vi "2B_Tech Serial Data Recording & DECADE 3.1.vi"() -> ()   [LabVIEW 2014]
uses:
  <vilib>/Instr/_visa.llb/VISA Set IO Buffer Mask.ctl
  <vilib>/Instr/_visa.llb/VISA Flush IO Buffer Mask.ctl
  <vilib>/Platform/TimedLoop/XDataNode/timing_clust.ctl
  <vilib>/Platform/TimedLoop/XDataNode/nitl_modes.ctl
  <vilib>/Platform/TimedLoop/XDataNode/wakeup.ctl
  C:/Program Files (x86)/National Instruments/LabVIEW 2014/examples/Data Communication/Network Streams/Simple Network Streams/support/Network Stream Command.ctl
  <vilib>/Utility/error.llb/whitespace.ctl
  <vilib>/Instr/_visa.llb/VISA Configure Serial Port (Instr).vi
  <vilib>/Utility/tcp.llb/UDP Multicast Write-Only Open.vi
  <vilib>/platform/TimedLoop/XDataNode/XDataNode.xnode
  <vilib>/Platform/TimedLoop/XDataNode/XDNodeRunTimeDep.lvlib
panel:
  out "SEPTIC TCP Error Out":errorcluster
  out "TCP packet\nSend to SEPTIC":bool
  in  "stop 2":bool
  out "FISH TCP Error Out":errorcluster
  out "TCP packet\nSend to FISH":bool
  in  "stop":bool
  out "Default file name":string
  out "error out":errorcluster
  out "Ambient/Cabin":bool
  out "Stop File Write":bool
  in  "timeout (10sec)":u32=3000
  in  "VISA resource name":refnum<visa-resource-name>="ASRL2::INSTR"
  out "Simulate 3 av":dbl
  out "Simulate\nConc":i32
  out "Simulate\nconc":bool
  out "3hr_alm_thresh":i32=80
  out "3hrAvg_Alarm":bool
  out "Inst_Alarm":bool
  out "Inst_alm_thresh":i32=220
  out "Time":string
  in  "Clear Display\nErrors":bool
  out "Read Error Counter\nfrom process loop":u32
  out "CABOZO UDP_ASCII_Out":string
  out "Ozo_array":string[](array[string])
  out "3hr_ozo_avg":dbl
  out "q_size":i32
  out "Data Output":string[](array[string])
  out "UDP packet\nSend status":bool
  out "TWBOZO UDP_ASCII_Out":string
  out "UDP_Out_Error":errorcluster
  out "UDP_Pack_num":u32
  out "Flight Number":string
  out "Number of times \nRead time out":u32
  out "Data Loop count":i32
  out "2B_Serial_error out":errorcluster
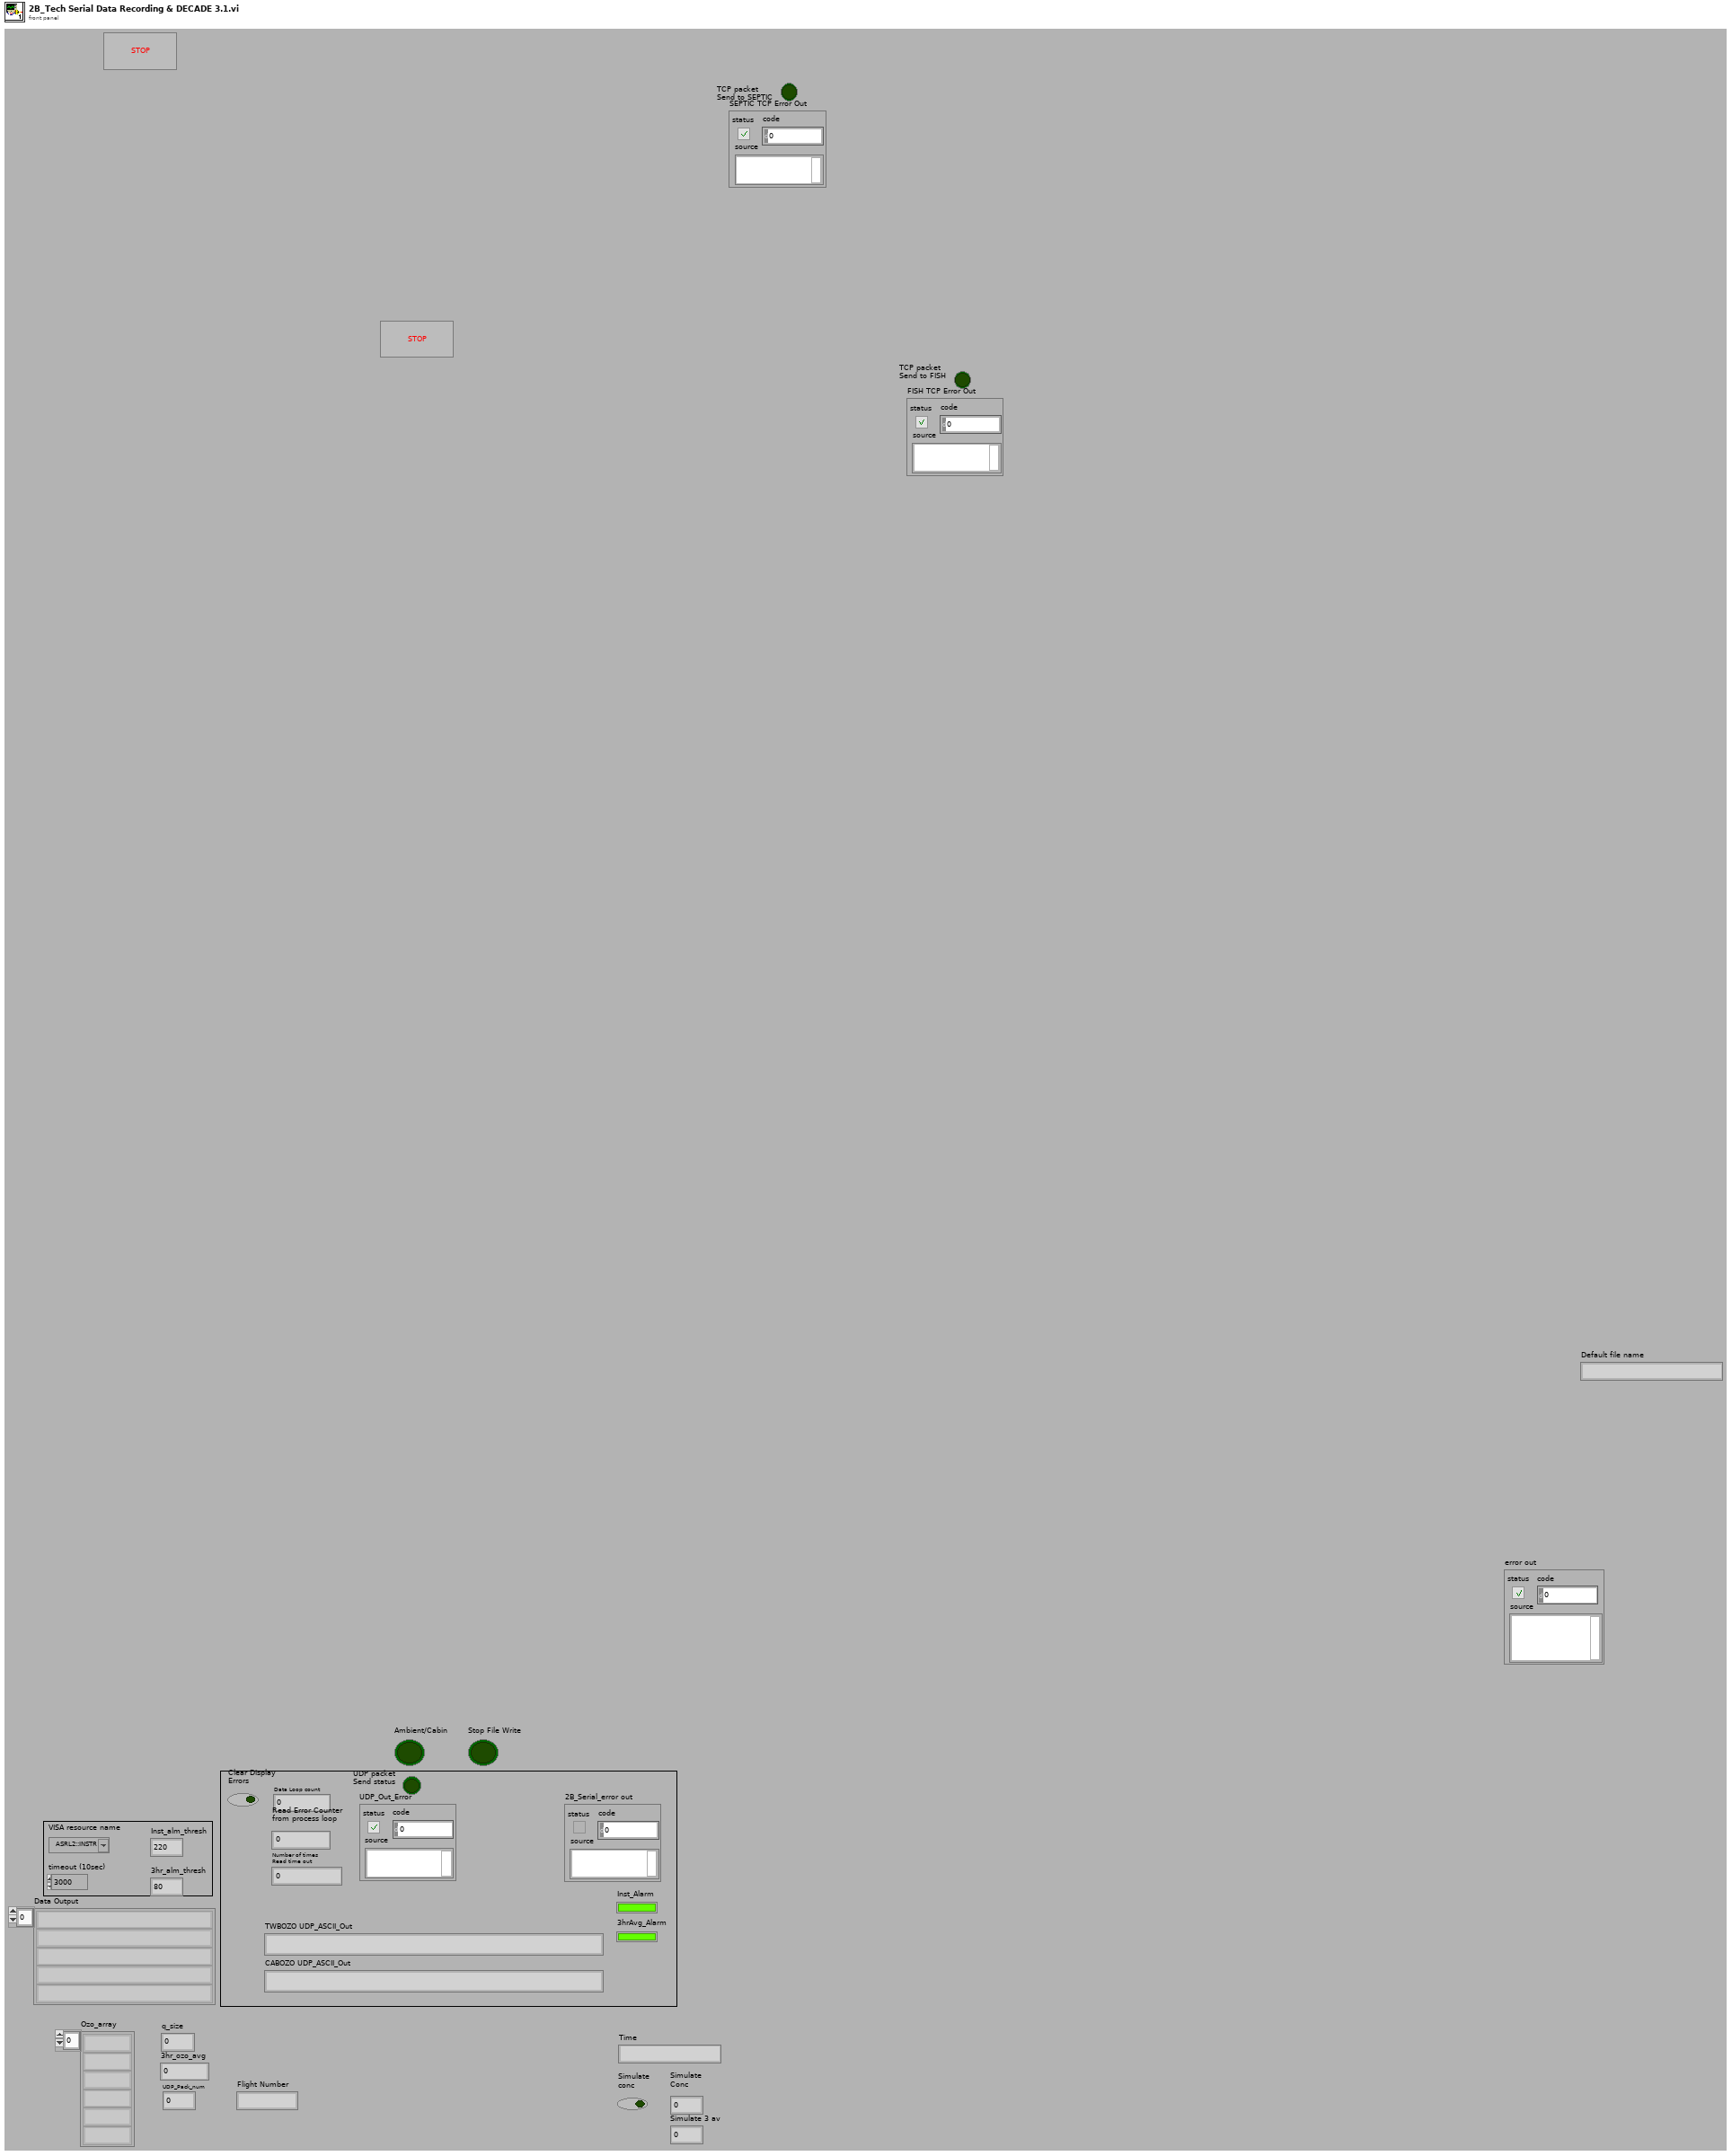
[diagram p1: front panel]
types:
  T1 = typedef "VISA Flush IO Buffer Mask.ctl" = u16
  T2 = typedef "VISA Set IO Buffer Mask.ctl" = u16
  T3 = typedef "XDNodeRunTimeDep.lvlib/timing_clust.ctl" = cluster{"Expected End [f-1]":u64, "Actual End [f-1]":u64, "Finished Late? [f-1]":bool, "Expected End [i-1]":u64, "Actual End [i-1]":u64, "Finished Late? [i-1]":bool, "Expected Start [i]":u64, "Actual Start [i]":u64, "Expected Start [f]":u64, "Actual Start [f]":u64, "Source Name":string, "Structure Name":string, "Period":i64, "Deadline":i64, "Offset":i64, "Start":i64, "Priority":i32, "Timeout":i32, "Mode":T4, "Wakeup Reason":T5, "Error":errorcluster, "Source Type":string, "Secondary Source Type":string, "Global End Time":u64, "Global Start Time":u64, "Frame Duration":u64, "Iteration Duration":u64, "Assigned CPU":i32, "I/O Scan Engine Mode":u32}
  T4 = typedef "XDNodeRunTimeDep.lvlib/nitl_modes.ctl" = enum32{"No Change", "Process missed periods, maintain original phase", "Discard missed periods, maintain original phase", "Process missed periods, ignore original phase", "Discard missed periods, ignore original phase"}
  T5 = typedef "XDNodeRunTimeDep.lvlib/wakeup.ctl" = enum32{"Normal", "Aborted", "Asynchronous wakeup", "Timing source error", "Timed loop error", "Timeout"}
  T6 = typedef "Network Stream Command.ctl" = cluster{"Message":string, "Message Data":variant}
  T7 = enum16{"open", "replace", "create", "open or create", "replace or create", "replace or create with confirmation"}
  T8 = typedef "whitespace.ctl" = u16
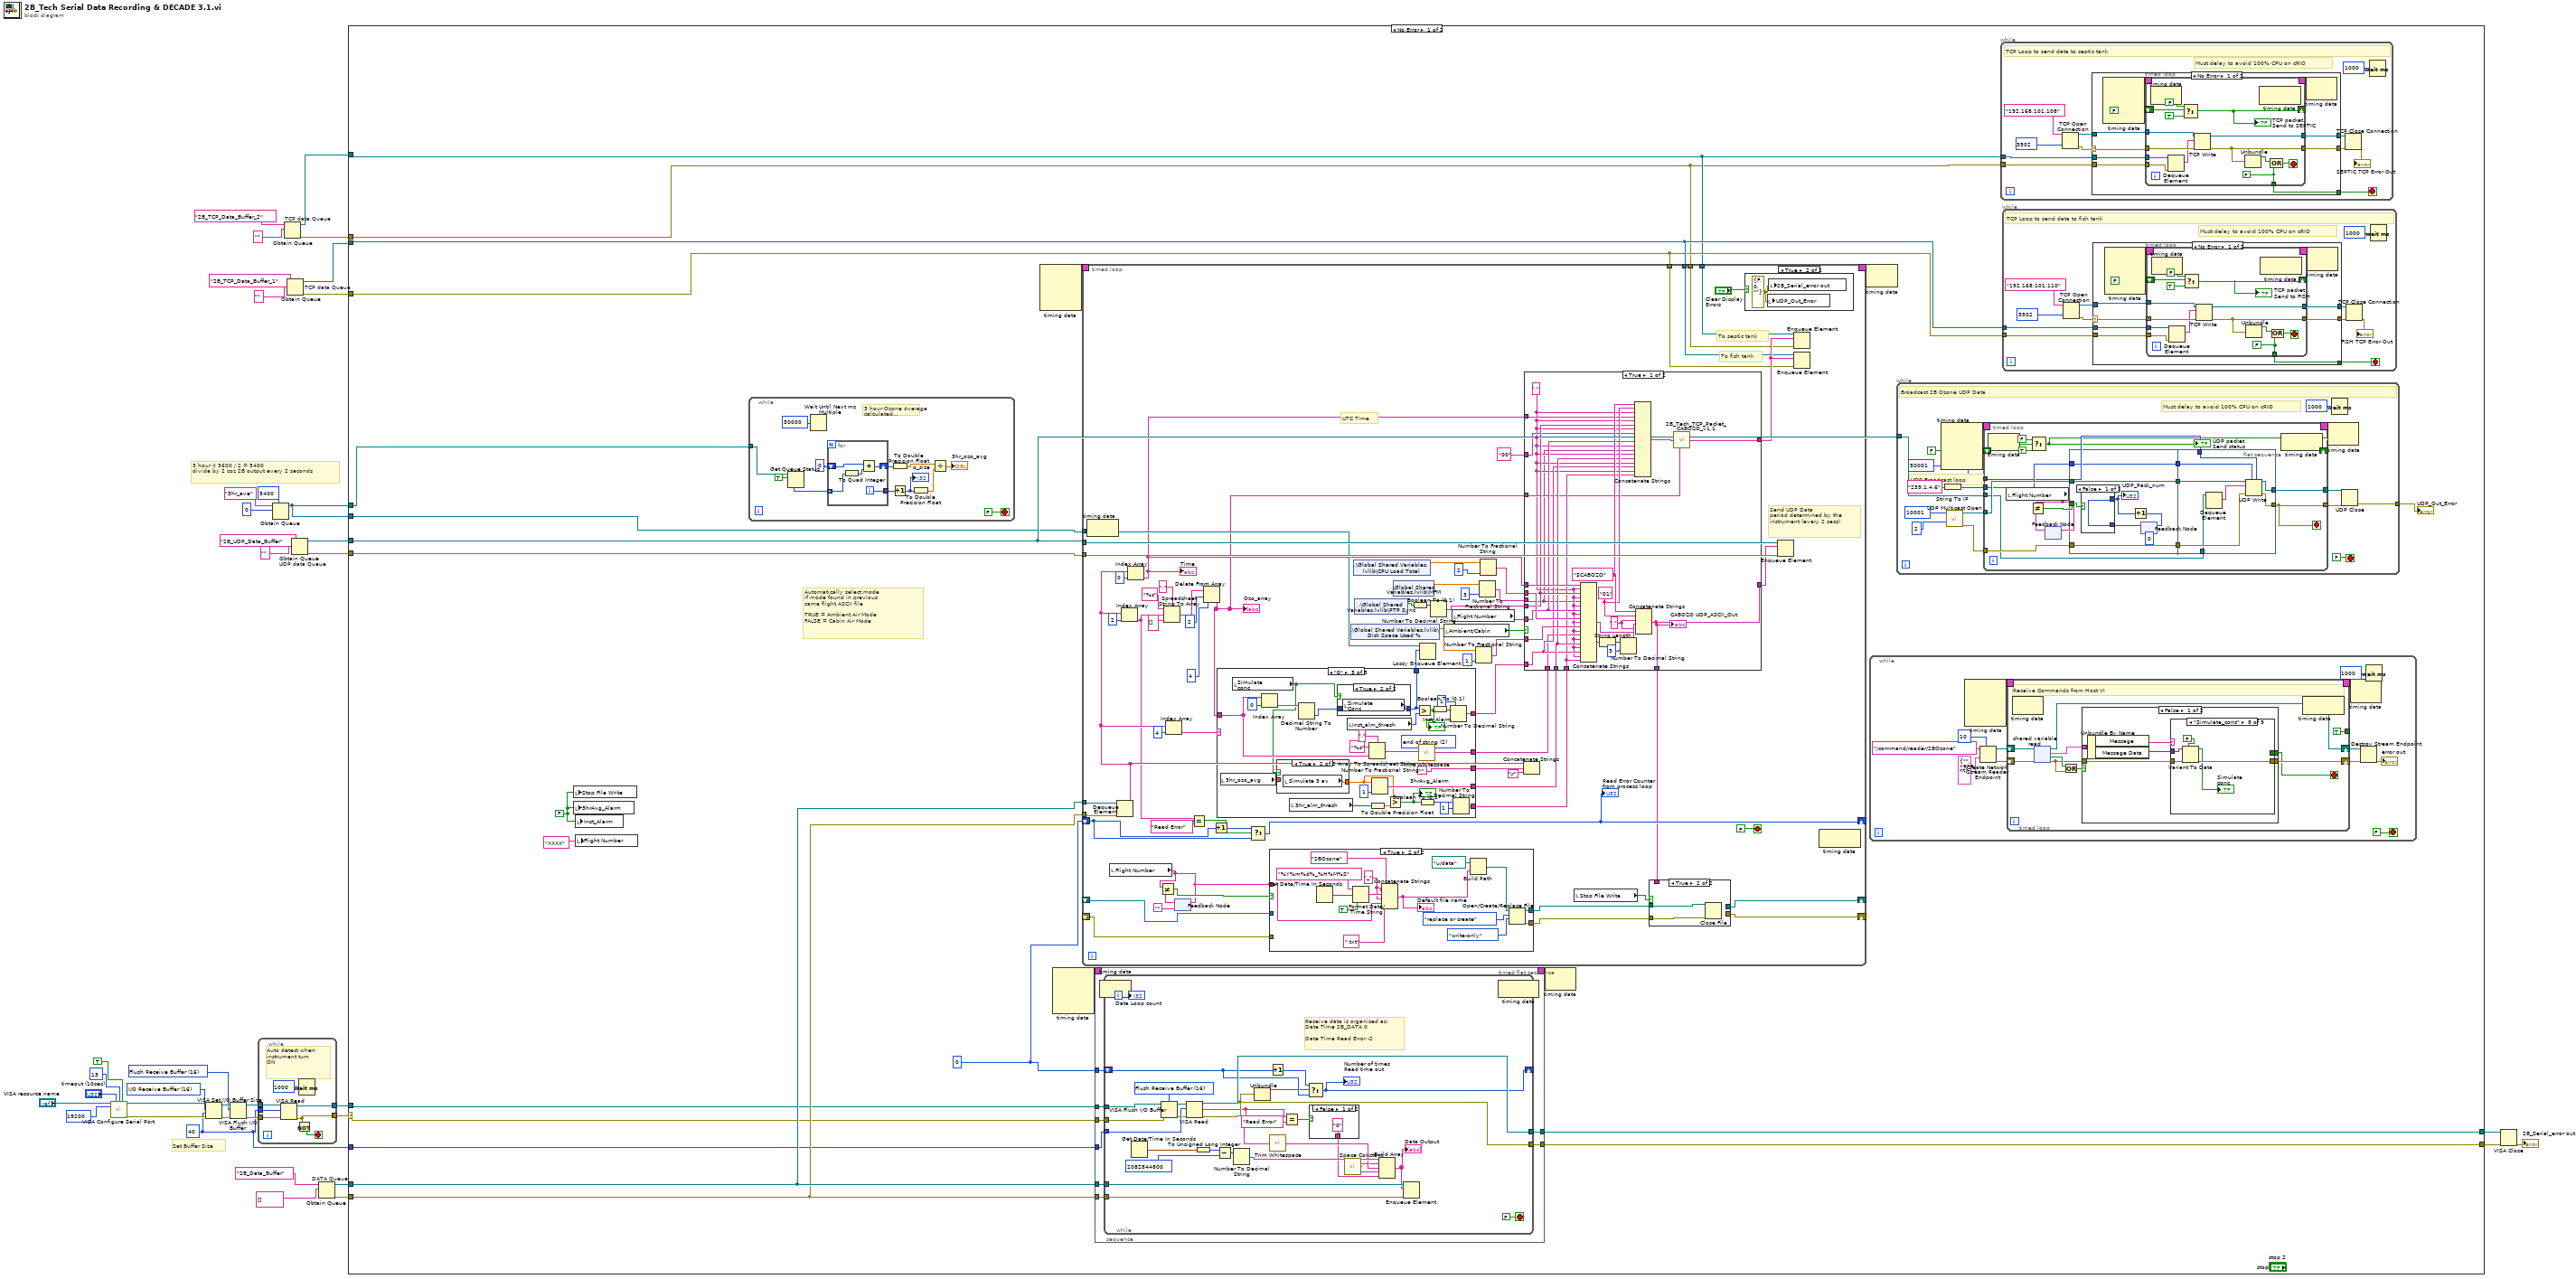
[diagram p0: block diagram]
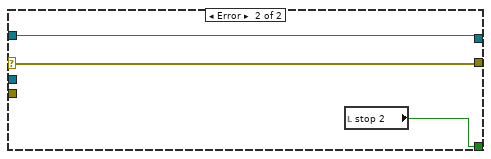
[diagram p2: hidden frame]
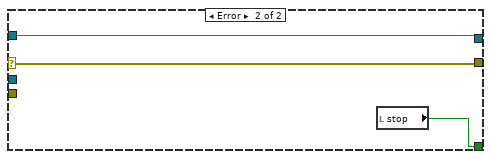
[diagram p3: hidden frame]
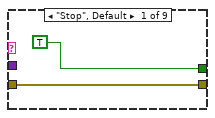
[diagram p4: hidden frame]
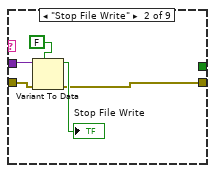
[diagram p5: hidden frame]
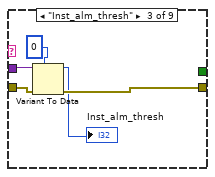
[diagram p6: hidden frame]
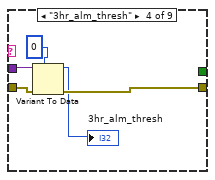
[diagram p7: hidden frame]
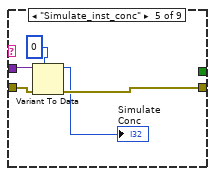
[diagram p8: hidden frame]
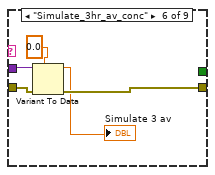
[diagram p9: hidden frame]
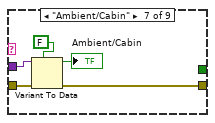
[diagram p10: hidden frame]
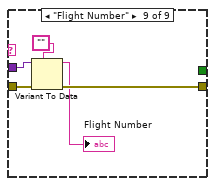
[diagram p11: hidden frame]
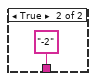
[diagram p13: hidden frame]
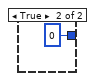
[diagram p14: hidden frame]
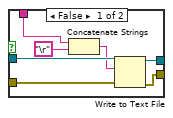
[diagram p15: hidden frame]
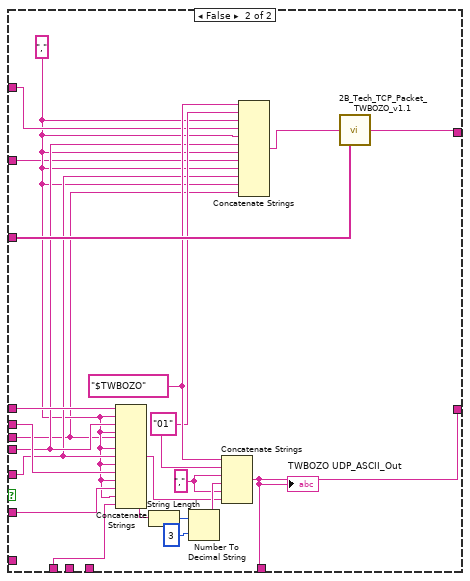
[diagram p18: hidden frame]
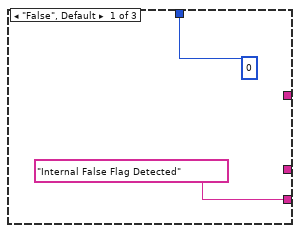
[diagram p19: hidden frame]
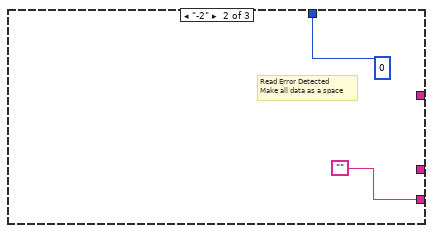
[diagram p20: hidden frame]
diagram:
  w9 = u32 40 ("size (4096)")
  w16 = T1 16 items=["Flush Receive Buffer"=16, "Write Transmit Buffer to Device"=32, "Flush Receive Buffer (No I/O)"=64, "Flush Transmit Buffer"=128] ("Mask")
  w17 = T2 16 items=["I/O Receive Buffer"=16, "I/O Transmit Buffer"=32, "I/O Receive and Transmit Buffer"=48] ("Mask")
  # "Set Buffer Size"
  # "3 hour X 3600 / 2 = 5400\ndivide by 2 coz 2B output every 2 seconds"
  n1 = call-poly "VISA Configure Serial Port"("VISA resource name"="VISA resource name", "timeout (10sec)"="timeout (10sec)", "termination char\n(0xA = '\\n' = LF)"=u8 13 ("termination char\n(0xA = '\\n' = LF)"), "Enable Termination\nChar (T)"=TRUE ("Enable Termination\nChar (T)"), "baud rate (9600)"=u32 19200) -> ("VISA resource name out"=w15:refnum<visa-resource-name>, "error out"=w14:errorcluster)  [unwired: 9 in]
  n2 = VISA Set I/O Buffer Size(VISA resource name=w15, mask (16)=w17, size (4096)=w9, error in (no error)=w14) -> (VISA resource name out=w18:refnum<visa-resource-name>, error out=w19:errorcluster)
  n3 = VISA Flush I/O Buffer(VISA resource name=w18, mask (16)=w16, error in (no error)=w19) -> (VISA resource name out=w13:refnum<visa-resource-name>, error out=w12:errorcluster)
  n4 = while {
    tunnel: w9 -> [w46]
    tunnel: w13 -> [w45]
    tunnel: w12 -> [w44]
    tunnel: [w42] -> w11
    tunnel: [w41] -> w10
    stop <- w43 stop-if-true
    # "Auto detect when\ninstrument turn\nON"
    n5 = VISA Read(VISA resource name=w45, byte count=w46, error in (no error)=w44) -> (VISA resource name out=w41:refnum<visa-resource-name>, error out=w42:errorcluster)  [unwired: 2 out]
    n6 = Not(x=w42) -> (.not. x?=w43:bool)
    n7 = Wait (ms)(milliseconds to wait=u32 1000) -> ()  [unwired: 1 out]
  }
  n8 = Obtain Queue(max queue size (-1, unlimited)=5400, name (unnamed)="3hr_ave", element data type=0 ("index")) -> (queue out=w25:refnum<queue>)  [unwired: 2 in, 2 out]
  n9 = Obtain Queue "TCP data Queue"(name (unnamed)="2B_TCP_Data_Buffer_2", element data type="") -> (queue out=w2:refnum<queue>, error out=w1:errorcluster)  [unwired: 3 in, 1 out]
  n10 = Obtain Queue "TCP data Queue"(name (unnamed)="2B_TCP_Data_Buffer_1", element data type="") -> (queue out=w4:refnum<queue>, error out=w3:errorcluster)  [unwired: 3 in, 1 out]
  n11 = Obtain Queue "UDP data Queue"(name (unnamed)="2B_UDP_Data_Buffer", element data type="") -> (queue out=w31:refnum<queue>, error out=w30:errorcluster)  [unwired: 3 in, 1 out]
  n12 = Obtain Queue "DATA Queue"(name (unnamed)="2B_Data_Buffer", element data type=string[] []) -> (queue out=w35:refnum<queue>, error out=w34:errorcluster)  [unwired: 3 in, 1 out]
  n13 = case shown="No Error" w11 {
    selector: w11 -> [w56 w529]
    tunnel: w10 -> [w57 w530]
    tunnel: [w69 w530] -> w38
    tunnel: [w61 w529] -> w39
    tunnel: w35 -> [w68 _]
    tunnel: w34 -> [w67 _]
    tunnel: w31 -> [w65 _]
    tunnel: w30 -> [w66 _]
    tunnel: w25 -> [w64 _]
    tunnel: w25 -> [w63 _]
    tunnel: w9 -> [w55 _]
    tunnel: w4 -> [w50 _]
    tunnel: w3 -> [w49 _]
    tunnel: w2 -> [w48 _]
    tunnel: w1 -> [w47 _]
    frame No Error {
      w52 = FALSE
      w62 = u32 0
      # "Automatically select mode\nif mode found in previous\nsame flight ASCII file\n\nTRUE = Ambient Air Mode\nFALSE = Cabin Air Mode"
      n14 = local write "Stop File Write"(w52) -> ()
      n15 = local write "3hrAvg_Alarm"(w52) -> ()
      n16 = local write "Inst_Alarm"(w52) -> ()
      n17 = local write "Flight Number"("XXXX" ("Flight Number")) -> ()
      n18 = while {
        tunnel: w64 -> [w284]
        stop <- FALSE stop-if-true
        # "3 hour Ozone Average calculated\nevery 30 seconds"
        n19 = Get Queue Status(queue=w284, return elements? (F)=TRUE) -> (elements=w281:i32[])  [unwired: 1 in, 7 out]
        n20 = Wait Until Next ms Multiple(millisecond multiple=u32 30000) -> ()  [unwired: 1 out]
        n21 = for {
          tunnel: [w296] -> w291
          shift-right: [w295] -> w289
          shift-left: i64 0 -> [w294]
          tunnel: w281 -> [w292] mode=indexing
          i -> [w296]
          n22 = To Quad Integer(1:w292) -> (0:w293:i64)
          n23 = Add(x=w294, y=w293) -> (x+y=w295:i64)
        }
        n24 = Increment(x=w291) -> (x+1=w285:i32)
        "q_size" <- w285
        n25 = To Double Precision Float(number=w289) -> (double precision float=w287:dbl)
        n26 = To Double Precision Float(number=w285) -> (double precision float=w288:dbl)
        n27 = Divide(x=w287, y=w288) -> (x/y=→"3hr_ozo_avg":dbl)
      }
      n28 = node-c288() -> (w60:T3)  [unwired: 4 in]
      n29 = node-c288() -> (w54:T3)  [unwired: 4 in]
      n30 = timed-loop {
        timing: w60 -> [_]
        timing-out: [_] -> w59
        tunnel: w68 -> [w417]
        tunnel: w67 -> [w416]
        tunnel: w65 -> [w415]
        tunnel: w66 -> [w414]
        tunnel: w63 -> [w388]
        shift-right: [w392] -> _
        shift-left: w62 -> [w393]
        shift-right: [w381] -> _
        shift-left: _ -> [w377]
        shift-right: [w375] -> _
        shift-left: _ -> [w376]
        tunnel: w50 -> [w357]
        tunnel: w49 -> [w356]
        tunnel: w48 -> [w355]
        tunnel: w47 -> [w354]
        stop <- FALSE stop-if-true
        # "UTC Time"
        # "To fish tank"
        # "To septic tank"
        # "Send UDP Data\nperiod determined by the\ninstrument (every 2 secs)"
        n31 = node-c288() -> ()  [unwired: 1 in, 1 out]
        n32 = local read "Flight Number"() -> (w373:string)
        n33 = Dequeue Element(queue=w417, error in (no error)=w416) -> (element=w401:string[])  [unwired: 1 in, 3 out]
        n34 = Index Array(array=w401, index=2) -> (element=w394:string)
        n35 = Index Array(array=w401, index=0) -> (element=w352:string)
        "Time" <- w352
        n36 = Spreadsheet String To Array(delimiter (Tab)=",", format string="%s", spreadsheet string=w394, array type (2D Dbl)=string[] [] ("Values Array")) -> (array=w406:string[])
        n37 = Index Array(array=w401, index=4) -> (element=w407:string)
        n38 = feedback #1("" ("Flight Number")) -> (w383:string)
        n39 = Not Equal?(x=w373, y=w383) -> (x != y?=w374:bool)
        n40 = feedback-in #1(w373) -> ()
        n41 = Equal?(x=w394, y="Read Error") -> (x = y?=w396:bool)
        n42 = Delete From Array(array=w406, length=2, index=4) -> (array with subset deleted=w359:string[])  [unwired: 1 out]
        "Ozo_array" <- w359
        n43 = Increment(x=w393) -> (x+1=w395:u32)
        n44 = case shown="\"0\"" w407 {
          tunnel: w359 -> [_ _ w513]
          tunnel: [_ _ w516] -> w402
          tunnel: [0 0 w501] -> w387
          tunnel: ["Internal False Flag Detected" "" ""] -> w400
          tunnel: [_ _ w510] -> w398
          tunnel: [_ _ w507] -> w390
          tunnel: [_ _ w503] -> w389
          frame "False", Default {
          }
          frame "-2" {
            # "Read Error Detected\nMake all data as a space"
          }
          frame "0" {
            w517 = T8 2 items=["both", "start of string", "end of string"] ("location (both)")
            n45 = local read "3hr_ozo_avg"() -> (w500:dbl)
            n46 = local read "Simulate\nconc"() -> (w496:bool)
            n47 = Index Array(array=w513, index=0) -> (element=w514:string)
            n48 = case shown="True" w496 {
              tunnel: [w521 w522] -> w499
              tunnel: w500 -> [w521 _]
              frame False {
              }
              frame True {
                n49 = local read "Simulate 3 av"() -> (w522:dbl)
              }
            }
            n50 = local read "3hr_alm_thresh"() -> (w497:i32)
            n51 = Decimal String To Number(string=w514) -> (number=w502:i32)  [unwired: 2 in, 1 out]
            n52 = case shown="True" w496 {
              tunnel: [w523 w524] -> w501
              tunnel: w502 -> [w523 _]
              frame False {
              }
              frame True {
                n53 = local read "Simulate\nConc"() -> (w524:i32)
              }
            }
            n54 = local read "Inst_alm_thresh"() -> (w498:i32)
            n55 = Array To Spreadsheet String(delimiter (Tab)=",", array=w513, 3:"%s" ("format string")) -> (spreadsheet string=w518:string)
            n56 = To Double Precision Float(number=w497) -> (double precision float=w504:dbl)
            n57 = Number To Fractional String(number=w499, precision (6)=i16 1) -> (F-format string=w510:string)  [unwired: 2 in]
            n58 = Greater?(x=w499, y=w504) -> (0:w505:bool)
            "3hrAvg_Alarm" <- w505
            n59 = Greater?(x=w501, y=w498) -> (0:w508:bool)
            "Inst_Alarm" <- w508
            n60 = call <vilib>:"Trim Whitespace.vi"("string"=w518, "location (both)"=w517) -> ("trimmed string"=w516:string)
            n61 = Boolean To (0,1)(Boolean=w505) -> (0, 1=w506:i16)
            n62 = Boolean To (0,1)(Boolean=w508) -> (0, 1=w509:i16)
            n63 = Number To Decimal String(number=w509, width (-)=i16 1) -> (decimal integer string=w507:string)
            n64 = Number To Decimal String(number=w506, width (-)=i16 1) -> (decimal integer string=w503:string)
          }
        }
        n65 = Select(t=w395, s=w396, f=w393) -> (s? t:f=w392:u32)
        "Read Error Counter\nfrom process loop" <- w392
        n66 = case shown="True" w374 {
          tunnel: [w428 w431] -> w379
          tunnel: [w427 w430] -> w378
          tunnel: w377 -> [w428 _]
          tunnel: w376 -> [w427 _]
          tunnel: w373 -> [_ w429]
          frame False {
          }
          frame True {
            w438 = "_" ("string")
            n67 = Get Date/Time In Seconds() -> (seconds since 1Jan1904=w439:timestamp)
            n68 = Format Date/Time String(time format string (%c)="%Y%m%d%_%H%M%S", seconds (now)=w439, UTC format=TRUE) -> (date/time string=w442:string)
            n69 = Concatenate Strings("2BOzone" ("string"), w438, w442, w438, w429, ".txt" ("string")) -> (w436:string)
            "Default file name" <- w436
            n70 = Build Path(base path=path "u:/data", name or relative path=w436) -> (appended path=w432:path)
            n71 = Open/Create/Replace File(file path (use dialog)=w432, operation (0:open)=T7."replace or create", access (0:read/write)=enum16{"read/write", "read-only", "write-only"}."write-only") -> (refnum out=w431:refnum<file>, error out=w430:errorcluster)  [unwired: 3 in, 1 out]
          }
        }
        n72 = shared-variable ".\\Global Shared Variables.lvlib\\Disk Space Used %"() -> (w361:dbl)  [unwired: 1 in, 1 out]
        n73 = shared-variable ".\\Global Shared Variables.lvlib\\CPU Load Total"() -> (w371:dbl)  [unwired: 1 in, 1 out]
        n74 = shared-variable ".\\Global Shared Variables.lvlib\\PTP Sync"() -> (w364:bool)  [unwired: 1 in, 1 out]
        n75 = shared-variable ".\\Global Shared Variables.lvlib\\MFM"() -> (w369:dbl)  [unwired: 1 in, 1 out]
        n76 = Boolean To (0,1)(Boolean=w364) -> (0, 1=w365:i16)
        n77 = Lossy Enqueue Element(queue=w388, element=w387) -> ()  [unwired: 1 in, 4 out]
        n78 = Number To Decimal String(number=w365) -> (decimal integer string=w363:string)  [unwired: 1 in]
        n79 = local read "Ambient/Cabin"() -> (w384:bool)
        n80 = local read "Flight Number"() -> (w385:string)
        n81 = Number To Fractional String(number=w361, precision (6)=i16 1) -> (F-format string=w360:string)  [unwired: 2 in]
        n82 = Number To Fractional String(number=w369, precision (6)=i16 3) -> (F-format string=w366:string)  [unwired: 2 in]
        n83 = Number To Fractional String(number=w371, precision (6)=i16 2) -> (F-format string=w370:string)  [unwired: 2 in]
        n84 = Concatenate Strings(w401, w400, "\r") -> ()  [unwired: 1 out]
        n85 = case shown="True" w384 {
          tunnel: [w462 w483] -> w413
          tunnel: w352 -> [w463 w484]
          tunnel: w402 -> [w451 w480]
          tunnel: w370 -> [w461 w482]
          tunnel: w366 -> [w445 w469]
          tunnel: w385 -> [w455 w474]
          tunnel: w398 -> [w454 _]
          tunnel: w390 -> [w453 _]
          tunnel: w389 -> [w452 _]
          tunnel: [w462 w483] -> w372
          tunnel: w363 -> [w456 w475]
          tunnel: w360 -> [w460 w481]
          tunnel: w352 -> [w457 w476]
          tunnel: w359 -> [w448 w479]
          tunnel: [w449 w471] -> w358
          tunnel: "00" -> [w447 w470]
          frame True {
            w446 = ","
            w458 = "01"
            w465 = ","
            w459 = "$CABOZO"
            n86 = Concatenate Strings(w463, w446, w456, w446, w445, w446, w455, w446, w461, w446, w460, w446, w451, w446, w454, w446, w453, w446, w452) -> (w464:string)
            n87 = String Length(string=w464) -> (length=w468:i32)
            n88 = Number To Decimal String(number=w468, width (-)=i16 3) -> (decimal integer string=w466:string)
            n89 = Concatenate Strings(w459, w458, w446, w457, w446, w456, w446, w447, w446, w455, w446, w445, w446, w454, w446, w453, w446, w452) -> (w450:string)
            n90 = Concatenate Strings(w459, w458, w465, w466, w465, w464) -> (w462:string)
            "CABOZO UDP_ASCII_Out" <- w462
            n91 = call "2B_Tech_TCP_Packet_CABOZO_v1.1.vi"("TCP Packet In"=w450, "Data Array"=w448) -> ("TCP Binary Packet"=w449:string)  [unwired: 13 in]
          }
          frame False {
            w473 = ","
            w477 = "01"
            w486 = ","
            w478 = "$TWBOZO"
            n92 = Concatenate Strings(w484, w473, w475, w473, w469, w473, w474, w473, w482, w473, w481, w473, w480) -> (w485:string)
            n93 = String Length(string=w485) -> (length=w489:i32)
            n94 = Number To Decimal String(number=w489, width (-)=i16 3) -> (decimal integer string=w487:string)
            n95 = Concatenate Strings(w478, w477, w486, w487, w486, w485) -> (w483:string)
            "TWBOZO UDP_ASCII_Out" <- w483
            n96 = Concatenate Strings(w478, w477, w473, w476, w473, w475, w473, w470, w473, w474, w473, w469) -> (w472:string)
            n97 = call "2B_Tech_TCP_Packet_TWBOZO_v1.1.vi"("TCP Packet In"=w472, "Data Array"=w479) -> ("TCP Binary Packet"=w471:string)  [unwired: 13 in]
          }
        }
        n98 = local read "Stop File Write"() -> (w380:bool)
        n99 = case shown="True" w380 {
          tunnel: w379 -> [w424 w426]
          tunnel: w378 -> [w423 w425]
          tunnel: [w420 _] -> w381
          tunnel: [w419 _] -> w375
          tunnel: w372 -> [w418 _]
          frame False {
            n100 = Concatenate Strings(w418, "\r") -> (w421:string)
            n101 = Write to Text File(file (use dialog)=w424, text=w421, error in=w423) -> (refnum out=w420:refnum<file>, error out=w419:errorcluster)  [unwired: 2 out]
          }
          frame True {
            n102 = Close File(refnum=w426, error in=w425) -> ()  [unwired: 2 out]
          }
        }
        n103 = case shown="True" "Clear Display\nErrors" {
          frame False {
          }
          frame True {
            w444 = errorcluster {"status"=FALSE, "code"=0, "source"=""} ("UDP Error Out")
            n104 = local write "UDP_Out_Error"(w444) -> ()
            n105 = local write "2B_Serial_error out"(w444) -> ()
          }
        }
        n106 = Enqueue Element(queue=w415, element=w413, error in (no error)=w414) -> ()  [unwired: 1 in, 3 out]
        n107 = Enqueue Element(queue=w355, element=w358, error in (no error)=w354) -> ()  [unwired: 1 in, 3 out]
        n108 = Enqueue Element(queue=w357, element=w358, error in (no error)=w356) -> ()  [unwired: 1 in, 3 out]
        n109 = node-c288() -> ()  [unwired: 1 in, 1 out]
      }
      n110 = timed-sequence {
        timing: w54 -> [_]
        timing-out: [_] -> w53
        tunnel: [w237] -> w69
        tunnel: w68 -> [w236]
        tunnel: w67 -> [w235]
        tunnel: w62 -> [w234]
        tunnel: [w233] -> w61
        tunnel: w57 -> [w232]
        tunnel: w56 -> [w231]
        tunnel: w55 -> [w230]
        n111 = timed-flat-sequence {
          tunnel: [w245] -> w237
          tunnel: w236 -> [w244]
          tunnel: w235 -> [w243]
          tunnel: w234 -> [w242]
          tunnel: [w241] -> w233
          tunnel: w232 -> [w240]
          tunnel: w231 -> [w239]
          tunnel: w230 -> [w238]
          n112 = node-c288() -> ()  [unwired: 1 in, 1 out]
          n113 = while {
            tunnel: [w264] -> w241
            shift-right: [w270] -> _
            shift-left: w242 -> [w271]
            tunnel: [w273] -> w245
            tunnel: w240 -> [w269]
            tunnel: w239 -> [w268]
            tunnel: w244 -> [w267]
            tunnel: w243 -> [w266]
            tunnel: w238 -> [w265]
            i -> [w272]
            stop <- FALSE stop-if-true
            w249 = T1 16 items=["Flush Receive Buffer"=16, "Write Transmit Buffer to Device"=32, "Flush Receive Buffer (No I/O)"=64, "Flush Transmit Buffer"=128] ("Mask")
            # "Receive data is organised as:\nDate Time 2B_DATA 0\n\nDate Time Read Error -2"
            n114 = Get Date/Time In Seconds() -> (seconds since 1Jan1904=w259:timestamp)
            n115 = VISA Flush I/O Buffer(VISA resource name=w269, mask (16)=w249, error in (no error)=w268) -> (VISA resource name out=w250:refnum<visa-resource-name>, error out=w248:errorcluster)
            n116 = VISA Read(VISA resource name=w250, byte count=w265, error in (no error)=w248) -> (VISA resource name out=w273:refnum<visa-resource-name>, read buffer=w247:string, error out=w264:errorcluster)  [unwired: 1 out]
            n117 = To Unsigned Long Integer(number=w259) -> (unsigned 32bit integer=w261:u32)
            n118 = Subtract(x=w261, y=u32 2082844800) -> (x-y=w258:u32)
            n119 = Number To Decimal String(number=w258) -> (decimal integer string=w255:string)  [unwired: 1 in]
            n120 = Unbundle(w264) -> ("status"=w262:bool)  [unwired: 2 out]
            n121 = Increment(x=w271) -> (x+1=w263:u32)
            n122 = call <vilib>:"Trim Whitespace.vi"("string"=w247) -> ("trimmed string"=w254:string)  [unwired: 1 in]
            n123 = Equal?(x=w247, y="Read Error") -> (x = y?=w256:bool)
            n124 = Select(t=w263, s=w262, f=w271) -> (s? t:f=w270:u32)
            "Number of times \nRead time out" <- w270
            n125 = case shown="False" w256 {
              tunnel: ["0" "-2"] -> w252
              frame False {
              }
              frame True {
              }
            }
            n126 = call <vilib>:"Space Constant.vi"() -> ("String"=w253:string)
            n127 = Build Array(w255, w253, w254, w253, w252) -> (w251:string[])
            "Data Output" <- w251
            n128 = Enqueue Element(queue=w267, element=w251, error in (no error)=w266) -> ()  [unwired: 1 in, 3 out]
            "Data Loop count" <- w272
          }
          n129 = node-c288() -> ()  [unwired: 1 in, 1 out]
        }
      }
      n130 = node-c288(w53) -> ()  [unwired: 1 out]
      n131 = node-c288(w59) -> ()  [unwired: 1 out]
      n132 = while {
        stop <- FALSE stop-if-true
        n133 = node-c288() -> (w155:T3)  [unwired: 4 in]
        n134 = Create Network Stream Reader Endpoint(7:10 ("reader buffer size"), 9:T6 {"Message"="", "Message Data"=variant} ("Message Cluster"), 11:"/command/reader/2BOzone" ("reader url")) -> (0:w161:errorcluster, 3:w162:refnum<k21>)  [unwired: 4 in]
        n135 = timed-loop "Host->Target Command Reader" {
          shift-right: [w172] -> w159
          shift-left: w161 -> [w175]
          shift-right: [w173] -> w158
          shift-left: w162 -> [w174]
          tunnel: [TRUE] -> _
          timing: w155 -> [_]
          timing-out: [_] -> w154
          stop <- w166 stop-if-true
          # "Receive Commands from Host VI"
          n136 = node-c288() -> ()  [unwired: 1 in, 1 out]
          n137 = shared-variable-read(w174, w175) -> (w173:refnum<k21>, w168:errorcluster, w170:bool, w171:T6)  [unwired: 1 in]
          n138 = Or(x=w170, y=w168) -> (x .or. y?=w169:bool)
          n139 = case shown="False" w169 {
            selector: w169 -> [_ w226]
            tunnel: w168 -> [w183 w227]
            tunnel: [w182 w227] -> w172
            tunnel: w171 -> [w180 _]
            tunnel: [w181 w226] -> w166
            frame False {
              n140 = Unbundle By Name(w180) -> ("Message"=w179:string, "Message Data"=w178:variant)
              n141 = case shown="\"Simulate_conc\"" w179 {
                tunnel: w183 -> [w185 w190 w195 w200 w205 w210 w215 w220 w225]
                tunnel: [w185 w186 w193 w198 w203 w208 w214 w219 w224] -> w182
                tunnel: w178 -> [_ w189 w194 w199 w204 w209 w213 w218 w223]
                tunnel: [TRUE _ _ _ _ _ _ _ _] -> w181
                frame "Stop", Default {
                }
                frame "Stop File Write" {
                  n142 = Variant To Data(error in=w190, type=FALSE, Variant=w189) -> (data=→"Stop File Write":bool, error out=w186:errorcluster)
                }
                frame "Inst_alm_thresh" {
                  n143 = Variant To Data(error in=w195, type=0, Variant=w194) -> (data=→"Inst_alm_thresh":i32, error out=w193:errorcluster)
                }
                frame "3hr_alm_thresh" {
                  n144 = Variant To Data(error in=w200, type=0, Variant=w199) -> (data=→"3hr_alm_thresh":i32, error out=w198:errorcluster)
                }
                frame "Simulate_inst_conc" {
                  n145 = Variant To Data(error in=w205, type=0, Variant=w204) -> (data=→"Simulate\nConc":i32, error out=w203:errorcluster)
                }
                frame "Simulate_3hr_av_conc" {
                  n146 = Variant To Data(error in=w210, type=0.0, Variant=w209) -> (data=→"Simulate 3 av":dbl, error out=w208:errorcluster)
                }
                frame "Ambient/Cabin" {
                  n147 = Variant To Data(error in=w215, type=FALSE, Variant=w213) -> (data=→"Ambient/Cabin":bool, error out=w214:errorcluster)
                }
                frame "Simulate_conc" {
                  n148 = Variant To Data(error in=w220, type=FALSE, Variant=w218) -> (data=→"Simulate\nconc":bool, error out=w219:errorcluster)
                }
                frame "Flight Number" {
                  n149 = Variant To Data(error in=w225, type="", Variant=w223) -> (data=→"Flight Number":string, error out=w224:errorcluster)
                }
              }
            }
            frame True {
            }
          }
          n150 = node-c288() -> ()  [unwired: 1 in, 1 out]
        }
        n151 = node-c288(w154) -> ()  [unwired: 1 out]
        n152 = Destroy Stream Endpoint(8:w159, 11:w158) -> (0:→"error out":errorcluster)
        n153 = Wait (ms)(milliseconds to wait=u32 1000) -> ()  [unwired: 1 out]
      }
      n154 = while {
        tunnel: w65 -> [w300]
        tunnel: [w299] -> w58
        stop <- FALSE stop-if-true
        # "Must delay to avoid 100% CPU on cRIO"
        # "UDP Broadcast loop"
        # "Broadcast 2B Ozone UDP Data"
        n155 = node-c288() -> (w302:T3)  [unwired: 4 in]
        n156 = String To IP(1:"239.1.4.6" ("name")) -> (0:w304:u32)
        n157 = call-poly <vilib>:"UDP Multicast Open.vi"("time-to-live (1)"=u16 2, "port"=u16 10001) -> ("error out"=w311:errorcluster, "connection ID"=w312:refnum<k16>)  [unwired: 8 in]
        n158 = timed-loop {
          tunnel: w312 -> [w329]
          tunnel: w311 -> [w328]
          tunnel: [w317] -> w307
          shift-right: [w314] -> _
          shift-left: FALSE -> [w322]
          tunnel: [w313] -> w306
          tunnel: w304 -> [w319]
          tunnel: u16 50001 ("port or service name") -> [w318]
          timing: w302 -> [_]
          timing-out: [_] -> w301
          tunnel: w300 -> [w315]
          stop <- w313 stop-if-true
          n159 = node-c288() -> ()  [unwired: 1 in, 1 out]
          n160 = local read "Flight Number"() -> (w316:string)
          n161 = Select(t=FALSE, s=w322, f=TRUE) -> (s? t:f=w314:bool)
          "UDP packet\nSend status" <- w314
          n162 = feedback-in #2(w316) -> ()
          n163 = feedback #2() -> (w324:string)  [unwired: 1 in]
          n164 = Not Equal?(x=w316, y=w324) -> (x != y?=w323:bool)
          n165 = flat-sequence {
            tunnel: w319 -> [w337]
            tunnel: w328 -> [w338]
            tunnel: w329 -> [w339]
            tunnel: [w339] -> w327
            tunnel: [w338] -> w326
            tunnel: [w337] -> w325
            tunnel: w323 -> [w336]
            tunnel: w318 -> [w349]
            tunnel: w327 -> [w348]
            tunnel: w326 -> [w347]
            tunnel: w325 -> [w346]
            tunnel: [w345] -> w317
            tunnel: [w344] -> w313
            tunnel: w315 -> [w342]
            frame #0 {
              n166 = feedback #3(u32 0) -> (w333:u32)
              n167 = case shown="False" w336 {
                tunnel: w333 -> [w340 _]
                tunnel: [w340 u32 0] -> w332
                frame False {
                }
                frame True {
                }
              }
              "UDP_Pack_num" <- w332
              n168 = Increment(x=w332) -> (x+1=w334:u32)
              n169 = feedback-in #3(w334) -> ()
            }
            frame #1 {
              n170 = Dequeue Element(queue=w342) -> (element=w343:string)  [unwired: 2 in, 3 out]
              n171 = UDP Write(address=w346, port or service name=w349, connection ID=w348, data in=w343, 8:w347) -> (error out=w344:errorcluster, 3:w345:refnum<k16>)  [unwired: 1 in]
            }
          }
          n172 = node-c288() -> ()  [unwired: 1 in, 1 out]
        }
        n173 = node-c288(w301) -> ()  [unwired: 1 out]
        n174 = Wait (ms)(milliseconds to wait=u32 1000) -> ()  [unwired: 1 out]
        n175 = UDP Close(connection ID=w307, 8:w306) -> (error out=w299:errorcluster)  [unwired: 1 out]
      }
      "UDP_Out_Error" <- w58
      n176 = while {
        tunnel: w47 -> [w72]
        tunnel: w48 -> [w71]
        stop <- w75 stop-if-true
        # "Must delay to avoid 100% CPU on cRIO"
        # "TCP Loop to send data to septic tank"
        n177 = TCP Open Connection(address="192.168.101.108", remote port or service name=u16 3502) -> (connection ID=w78:refnum<k5>, error out=w73:errorcluster)  [unwired: 3 in]
        n178 = case shown="No Error" w73 {
          selector: w73 -> [w83 w110]
          tunnel: w78 -> [w88 w111]
          tunnel: [w87 w111] -> w77
          tunnel: [w86 w110] -> w76
          tunnel: [w85 w109] -> w75
          tunnel: w71 -> [w82 _]
          tunnel: w72 -> [w81 _]
          frame No Error {
            n179 = node-c288() -> (w90:T3)  [unwired: 4 in]
            n180 = timed-loop {
              tunnel: w88 -> [w104]
              tunnel: w83 -> [w103]
              tunnel: [w102] -> w87
              tunnel: [w101] -> w86
              tunnel: [w91] -> w85
              shift-right: [w95] -> _
              shift-left: FALSE -> [w98]
              timing: w90 -> [_]
              timing-out: [_] -> w89
              tunnel: w82 -> [w94]
              tunnel: w81 -> [w93]
              stop <- w99 stop-if-true
              w91 = FALSE
              n181 = node-c288() -> ()  [unwired: 1 in, 1 out]
              n182 = Dequeue Element(queue=w94, error in (no error)=w93) -> (element=w92:string)  [unwired: 1 in, 3 out]
              n183 = Select(t=FALSE, s=w98, f=TRUE) -> (s? t:f=w95:bool)
              "TCP packet\nSend to SEPTIC" <- w95
              n184 = TCP Write(connection ID=w104, data in=w92, error in (no error)=w103) -> (connection ID out=w102:refnum<k5>, error out=w101:errorcluster)  [unwired: 1 in, 1 out]
              n185 = Unbundle(w101) -> ("status"=w100:bool)  [unwired: 2 out]
              n186 = node-c288() -> ()  [unwired: 1 in, 1 out]
              n187 = Compound Arithmetic op=OR(w100, w91) -> (w99:bool)
            }
            n188 = node-c288(w89) -> ()  [unwired: 1 out]
          }
          frame Error {
            n189 = local read "stop 2"() -> (w109:bool)
          }
        }
        n190 = TCP Close Connection(connection ID=w77, error in (no error)=w76) -> (error out=→"SEPTIC TCP Error Out":errorcluster)  [unwired: 1 in, 1 out]
        n191 = Wait (ms)(milliseconds to wait=u32 1000) -> ()  [unwired: 1 out]
      }
      n192 = while {
        tunnel: w50 -> [w114]
        tunnel: w49 -> [w113]
        stop <- w117 stop-if-true
        # "Must delay to avoid 100% CPU on cRIO"
        # "TCP Loop to send data to fish tank"
        n193 = TCP Open Connection(address="192.168.101.110", remote port or service name=u16 3502) -> (connection ID=w120:refnum<k5>, error out=w115:errorcluster)  [unwired: 3 in]
        n194 = case shown="No Error" w115 {
          selector: w115 -> [w125 w152]
          tunnel: w120 -> [w130 w153]
          tunnel: [w129 w153] -> w119
          tunnel: [w128 w152] -> w118
          tunnel: [w127 w151] -> w117
          tunnel: w114 -> [w124 _]
          tunnel: w113 -> [w123 _]
          frame No Error {
            n195 = node-c288() -> (w132:T3)  [unwired: 4 in]
            n196 = timed-loop {
              tunnel: w130 -> [w146]
              tunnel: w125 -> [w145]
              tunnel: [w144] -> w129
              tunnel: [w143] -> w128
              tunnel: [w140] -> w127
              shift-right: [w136] -> _
              shift-left: FALSE -> [w139]
              timing: w132 -> [_]
              timing-out: [_] -> w131
              tunnel: w124 -> [w135]
              tunnel: w123 -> [w134]
              stop <- w141 stop-if-true
              w140 = FALSE
              n197 = node-c288() -> ()  [unwired: 1 in, 1 out]
              n198 = Dequeue Element(queue=w135, error in (no error)=w134) -> (element=w133:string)  [unwired: 1 in, 3 out]
              n199 = Select(t=FALSE, s=w139, f=TRUE) -> (s? t:f=w136:bool)
              "TCP packet\nSend to FISH" <- w136
              n200 = TCP Write(connection ID=w146, data in=w133, error in (no error)=w145) -> (connection ID out=w144:refnum<k5>, error out=w143:errorcluster)  [unwired: 1 in, 1 out]
              n201 = Unbundle(w143) -> ("status"=w142:bool)  [unwired: 2 out]
              n202 = node-c288() -> ()  [unwired: 1 in, 1 out]
              n203 = Compound Arithmetic op=OR(w142, w140) -> (w141:bool)
            }
            n204 = node-c288(w131) -> ()  [unwired: 1 out]
          }
          frame Error {
            n205 = local read "stop"() -> (w151:bool)
          }
        }
        n206 = TCP Close Connection(connection ID=w119, error in (no error)=w118) -> (error out=→"FISH TCP Error Out":errorcluster)  [unwired: 1 in, 1 out]
        n207 = Wait (ms)(milliseconds to wait=u32 1000) -> ()  [unwired: 1 out]
      }
    }
    frame Error {
    }
  }
  n208 = VISA Close(VISA resource name=w38, error in (no error)=w39) -> (error out=→"2B_Serial_error out":errorcluster)
